vi "Denoising New.vi"(0 "Higher Cut-Off\nfor Highpass Filter":dbl=1.0, 1 "Lower Cut-Off\nfor Lowpass Filter":dbl=70.0, 2 "Array in":dbl[][](array[numeric]), 5 "Sampling Frequency\nfor  Bandpass Filtering":dbl=512.0, 8 "Absolute Data":bool) -> (7 "Array out":dbl[][](array[numeric]))   [LabVIEW 2023]
uses:
  <vilib>/Analysis/3filter.llb/Filter Passband Type.ctl
  <vilib>/Analysis/NI_AALBase.lvlib
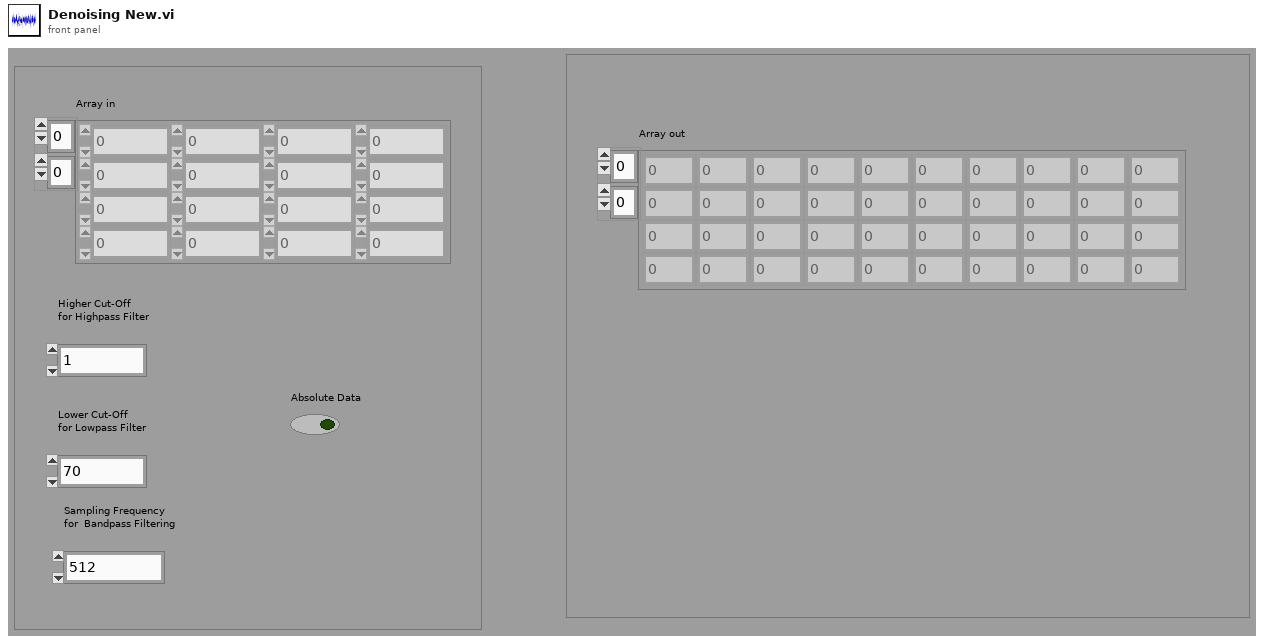
[diagram p1: front panel]
types:
  T1 = typedef "NI_AALBase.lvlib/Filter Passband Type.ctl" = enum32{"Lowpass", "Highpass", "Bandpass", "Bandstop"}
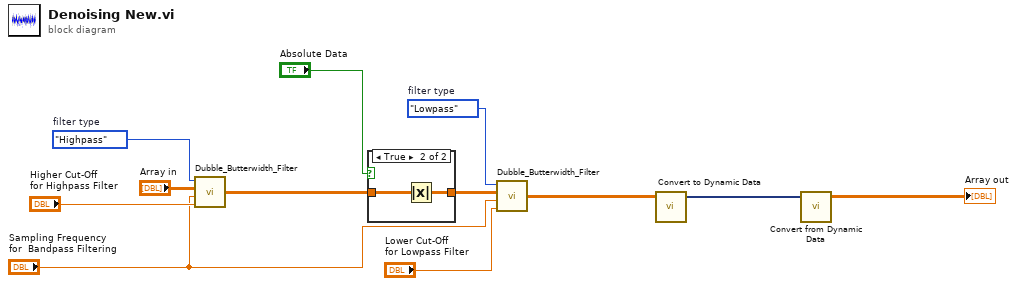
[diagram p0: block diagram]
diagram:
  w9 = Filter_Passband_Type."Lowpass"  # filter type
  w10 = Filter_Passband_Type."Highpass"  # filter type
  n1 = call "Dubble_Butterwidth_Filter.vi"("Higher Cut-Off"="Higher Cut-Off\nfor Highpass Filter", "sampling freq: fs"="Sampling Frequency\nfor  Bandpass Filtering", "Array in"="Array in", "filter type"=w10) -> ("Array out"=w11:dbl[][])
  n2 = case shown="True" "Absolute Data" {
    tunnel: w11 -> [w13 w15]
    tunnel: [w13 w14] -> w12
    frame False {
    }
    frame True {
      n3 = Absolute Value(x=w15) -> (abs(x)=w14:dbl[][])
    }
  }
  n4 = call "Dubble_Butterwidth_Filter.vi"("Higher Cut-Off"="Lower Cut-Off\nfor Lowpass Filter", "sampling freq: fs"="Sampling Frequency\nfor  Bandpass Filtering", "Array in"=w12, "filter type"=w9) -> ("Array out"=w8:dbl[][])
  n5 = call "Convert to Dynamic Data"("2D Array"=w8) -> ("Dynamic Data Type"=w7:dynamicdata)  [unwired: 3 in]
  n6 = call "Convert from Dynamic Data"("Dynamic Data Type"=w7) -> ("Array"=→"Array out":dbl[][])  [unwired: 3 in]
